vi "Set Field.vi"(1 "Rate":dbl=10.0, 2 "Field":dbl) -> ()   [LabVIEW 2013]
uses:
  PPMS Global.vi
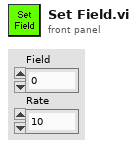
[diagram p1: front panel]
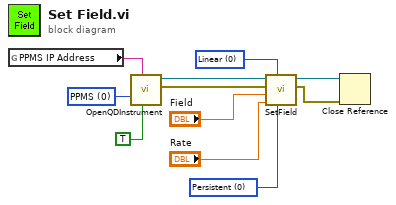
[diagram p0: block diagram]
diagram:
  w7 = 0 items=["Linear", "NoOvershoot", "Oscillate"] ("Approach")
  w8 = 0 items=["Persistent", "Driven"] ("Mode")
  w10 = 0 items=["PPMS", "VersaLab", "DynaCool", "SVSM"] ("Instrument\nType")
  n1 = global read "PPMS Global.vi" "PPMS IP Address"() -> (w9:string)
  n2 = call "OpenQDInstrument.vi"("Remote"=TRUE, "IP Address"=w9, "Instrument Type"=w10) -> ("error out"=w5:errorcluster, "Instrument Ref"=w6:refnum<k24>)  [unwired: 5 in]
  n3 = call "SetField.vi"("Mode"=w8, "Approach"=w7, "Rate"="Rate", "Field"="Field", "error in (no error)"=w5, "Instrument Ref In"=w6) -> ("error out"=w3:errorcluster, "Instrument Ref Out"=w4:refnum<k24>)  [unwired: 1 in, 1 out]
  n4 = Close Reference(reference=w4, error in (no error)=w3) -> ()  [unwired: 1 out]
